vi "高精度读.vi"(3 "串口号":refnum<visa-resource-name>) -> (1 "应答":string)   [LabVIEW 2012]
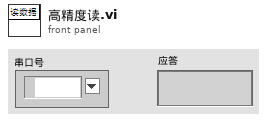
[diagram p1: front panel]
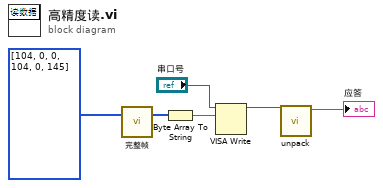
[diagram p0: block diagram]
diagram:
  n1 = call "完整帧.vi"("不完整帧"=u8[] [104, 0, 0, 104, 0, 145]) -> ("完整帧"=w1:u8[])  [unwired: 2 in]
  n2 = Byte Array To String(unsigned byte array=w1) -> (string=w2:string)
  n3 = VISA Write(VISA resource name="串口号", write buffer=w2) -> (VISA resource name out=w4:refnum<visa-resource-name>)  [unwired: 1 in, 2 out]
  n4 = call "unpack.vi"("串口号输入"=w4) -> ("应答"=→"应答":string)  [unwired: 5 in, 1 out]
